vi "WaveformComponent, Create One Phase.vi"(0 "waveform in":waveform(dbl)={"t0"=timestamp(3474853248.0780005 s since 1904-01-01), "dt"=1e-06, "Y"=[]}, 1 "phase parameters":T1={"offset"=0.5, "amplitude"=2.5, "delay"=0.00019999999999999998, "leading edge"=4.9999999999999996e-05, "pulse width"=0.00039999999999999996, "trailing edge"=7.5e-05, "ref level %"=33.3} {"ref level %" format="%.3f"; "offset" format="%.3f"; "pulse width" format="%.1f"; "trailing edge" format="%.1f"; "amplitude" format="%.3f"; "delay" format="%.1f"; "leading edge" format="%.1f"}) -> (3 "waveform out":waveform(dbl)(graph)={"t0"=timestamp(3474853248.0780005 s since 1904-01-01), "dt"=1e-06, "Y"=[]})   [LabVIEW 2010]
uses:
  Pulse Parameters.ctl
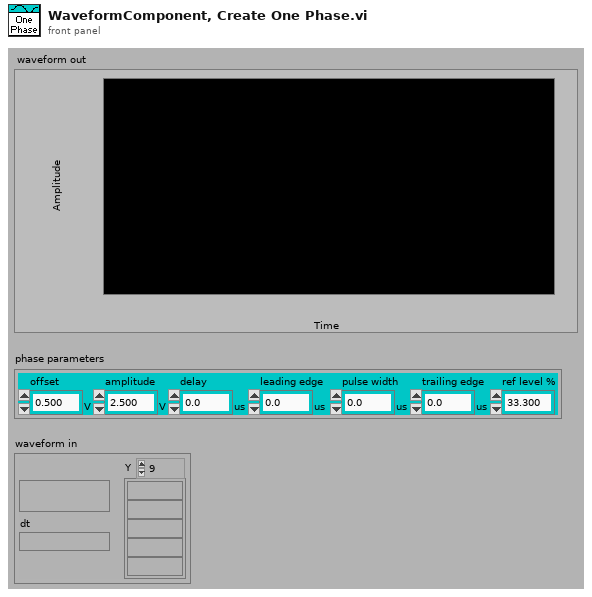
[diagram p1: front panel]
types:
  T1 = typedef "Pulse Parameters.ctl" = cluster{"offset":dbl[unit], "amplitude":dbl[unit], "delay":dbl[unit], "leading edge":dbl[unit], "pulse width":dbl[unit], "trailing edge":dbl[unit], "ref level %":dbl}
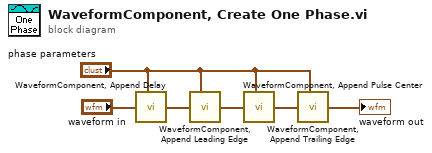
[diagram p0: block diagram]
diagram:
  n1 = call "WaveformComponent, Append Delay.vi"("waveform in"="waveform in", "append parameters"="phase parameters") -> ("waveform out"=w5:waveform(dbl))  [unwired: 1 in]
  n2 = call "WaveformComponent, Append Leading Edge.vi"("waveform in"=w5, "append parameters"="phase parameters") -> ("waveform out"=w4:waveform(dbl))  [unwired: 1 in]
  n3 = call "WaveformComponent, Append Pulse Center.vi"("waveform in"=w4, "append parameters"="phase parameters") -> ("waveform out"=w3:waveform(dbl))  [unwired: 1 in]
  n4 = call "WaveformComponent, Append Trailing Edge.vi"("waveform in"=w3, "append parameters"="phase parameters") -> ("waveform out"=→"waveform out":waveform(dbl))  [unwired: 1 in]
